vi "BRig_RT_comm_webdav_connect.vi"(8 "input_error":errorcluster, 10 "input_password":string, 11 "input_username":string="Paul Jonak") -> (0 "output_error":errorcluster, 2 "output_Iconnected":bool, 3 "output_hSession":T1, 4 "output_code":u8)   [LabVIEW 2014]
uses:
  <vilib>/WebDAVClient/Advanced/SessionHandle.ctl
  <vilib>/WebDAVClient/NI_WebDAV.lvlib
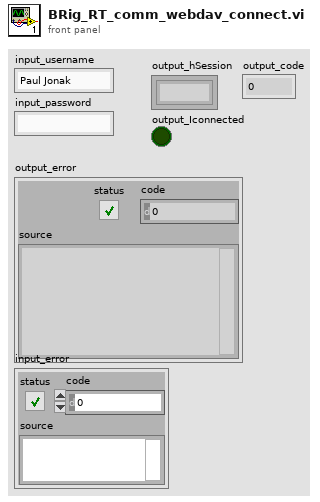
[diagram p1: front panel]
types:
  T1 = typedef "NI_WebDAV.lvlib/SessionHandle.ctl" = refnum<k1>
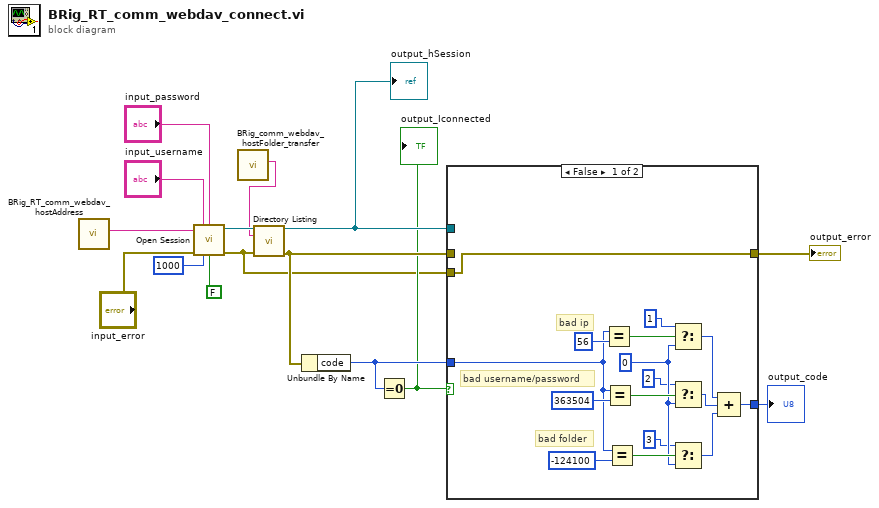
[diagram p0: block diagram]
diagram:
  n1 = call "BRig_RT_comm_webdav_hostAddress.vi"() -> ("output_HostAddress"=w4:string)  [unwired: 11 in]
  n2 = call <vilib>:"Open Session.vi"("host uri prefix"=w4, "username"="input_username", "password"="input_password", "error in (no error)"="input_error", "timeout ms"=1000, "verify server?"=FALSE) -> ("session handle out"=w14:T1, "error out"=w2:errorcluster)  [unwired: 8 in]
  n3 = call "BRig_comm_webdav_hostFolder_transfer.vi"() -> ("output_HostFolder"=w5:string)  [unwired: 11 in]
  n4 = call <vilib>:"Directory Listing.vi"("session handle"=w14, "relative uri"=w5, "error in (no error)"=w2) -> ("session handle out"=w11:T1, "error out"=w10:errorcluster)  [unwired: 9 in, 2 out]
  "output_hSession" <- w11
  n5 = Unbundle By Name(w10) -> ("code"=w8:i32)
  n6 = Equal To 0?(x=w8) -> (x = 0?=w7:bool)
  "output_Iconnected" <- w7
  n7 = case shown="False" w7 {
    tunnel: w8 -> [w28 _]
    tunnel: w11 -> [_ _]
    tunnel: w10 -> [_ w32]
    tunnel: [w18 _] -> w9
    tunnel: [w16 w32] -> w3
    tunnel: w2 -> [w16 _]
    frame False {
      w24 = u8 0
      # "bad folder"
      # "bad username/password"
      # "bad ip"
      n8 = Equal?(x=w28, y=56) -> (x = y?=w27:bool)
      n9 = Equal?(x=w28, y=363504) -> (x = y?=w26:bool)
      n10 = Equal?(x=w28, y=-124100) -> (x = y?=w25:bool)
      n11 = Select(t=u8 1, s=w27, f=w24) -> (s? t:f=w17:u8)
      n12 = Select(t=u8 2, s=w26, f=w24) -> (s? t:f=w20:u8)
      n13 = Select(t=u8 3, s=w25, f=w24) -> (s? t:f=w19:u8)
      n14 = Compound Arithmetic op=ADD(w17, w20, w19) -> (w18:u8)
    }
    frame True {
    }
  }
  "output_code" <- w9
  "output_error" <- w3
